vi "Query Heater Output 9620.vi"(8 "error in (no error)":errorcluster, 11 "VISA resource name":refnum<visa-resource-name>="COM3") -> (0 "error out":errorcluster, 2 "Current heater output":dbl, 3 "VISA resource name out":refnum<visa-resource-name>)   [LabVIEW 2017]
panel:
  out "read buffer 2":string
  out "Command string":string="S"
  out "read buffer":string
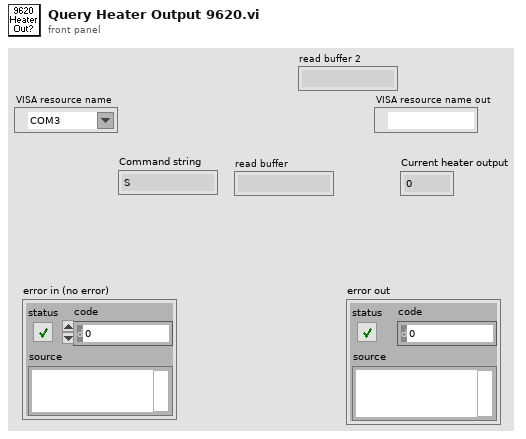
[diagram p1: front panel]
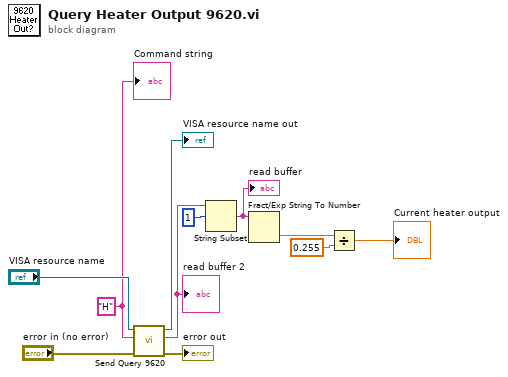
[diagram p0: block diagram]
diagram:
  w5 = "H"
  n1 = call "Send Query 9620.vi"("error in (no error)"="error in (no error)", "Query"=w5, "VISA resource name"="VISA resource name") -> ("error out"=→"error out":errorcluster, "read buffer"=w10:string, "VISA resource name out"=→"VISA resource name out":refnum<visa-resource-name>)  [unwired: 6 in]
  "read buffer 2" <- w10
  n2 = String Subset(string=w10, offset (0)=1) -> (substring=w4:string)  [unwired: 1 in]
  "read buffer" <- w4
  n3 = Fract/Exp String To Number(string=w4) -> (number=w2:dbl)  [unwired: 3 in, 1 out]
  n4 = Divide(x=w2, y=0.255) -> (x/y=→"Current heater output":dbl)
  "Command string" <- w5
